vi "配置初始化.vi"(8 "error in (no error)":errorcluster caption="错误输入（无错误）") -> (0 "error out":errorcluster)   [LabVIEW 2022 SP3, in "超标留样集成.lvlib"]
uses:
  DR803M4/DR803M4.lvlib
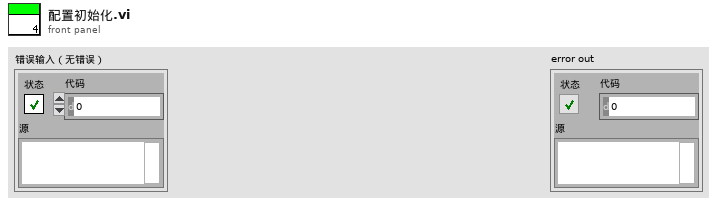
[diagram p1: front panel]
types:
  T1 = enum16{"德润DR803M", "德润DR803L", "德润DR803F", "科盛超标留样", "德润DR803M4", "ESTD1200"}
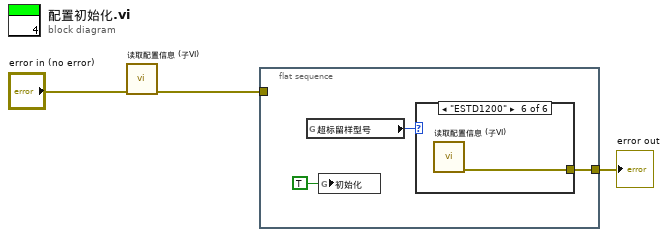
[diagram p0: block diagram]
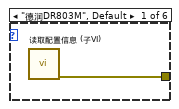
[diagram p2: hidden frame]
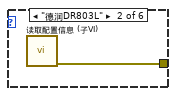
[diagram p3: hidden frame]
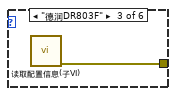
[diagram p4: hidden frame]
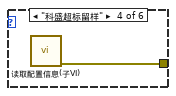
[diagram p5: hidden frame]
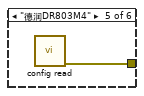
[diagram p6: hidden frame]
diagram:
  n1 = call "读取配置信息 (子VI).vi"("error in (no error)"="error in (no error)") -> ("错误输出"=w3:errorcluster)  [unwired: 10 in]
  n2 = flat-sequence {
    tunnel: w3 -> [_]
    tunnel: [w5] -> w1
    frame #0 {
      n3 = global read "断电保存全局.vi" "超标留样型号"() -> (w6:T1)
      n4 = global write "断电保存全局.vi" "初始化"(TRUE ("初始化")) -> ()
      n5 = case shown="\"ESTD1200\"" w6 {
        tunnel: [w7 w8 w9 w10 w11 w12] -> w5
        frame "德润DR803M", Default {
          n6 = call "读取配置信息 (子VI).vi"() -> ("错误输出"=w7:errorcluster)  [unwired: 11 in]
        }
        frame "德润DR803L" {
          n7 = call "读取配置信息 (子VI).vi"() -> ("错误输出"=w8:errorcluster)  [unwired: 11 in]
        }
        frame "德润DR803F" {
          n8 = call "读取配置信息(子VI).vi"() -> ("错误输出"=w9:errorcluster)  [unwired: 11 in]
        }
        frame "科盛超标留样" {
          n9 = call "读取配置信息(子VI).vi"() -> ("错误输出"=w10:errorcluster)  [unwired: 11 in]
        }
        frame "德润DR803M4" {
          n10 = call "config read.vi"() -> ("error out"=w11:errorcluster)  [unwired: 11 in]
        }
        frame "ESTD1200" {
          n11 = call "读取配置信息 (子VI).vi"() -> ("错误输出"=w12:errorcluster)  [unwired: 11 in]
        }
      }
    }
  }
  "error out" <- w1
